vi "Close.vi"(8 "error in (no error)":errorcluster, 11 "Sparkfun Atomic IMU in":refnum<class "Sparkfun Atomic IMU.lvclass">) -> (0 "error out":errorcluster)   [LabVIEW 2019, in "Sparkfun Atomic IMU.lvclass"]
doc: "Terminates the software connection to the sensor."
uses:
  Sparkfun Atomic IMU.lvclass
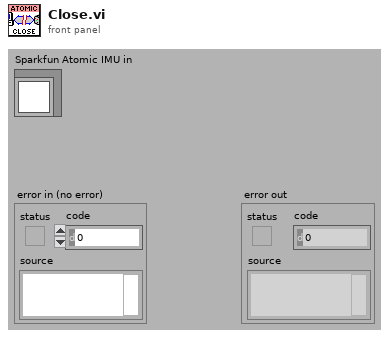
[diagram p1: front panel]
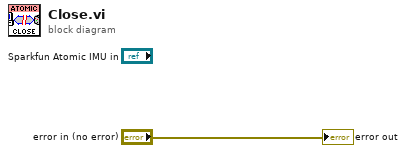
[diagram p0: block diagram]
diagram:
  "error out" <- "error in (no error)"
